vi "Main.vi"() -> ()   [LabVIEW 2023]
uses:
  3e66f978-0bac-48a9-bd70-621d12ad9d2c.vi
  <vilib>/JDP Science/JSONtext/JSON text to Variant.vi
  <vilib>/JDP Science/JSONtext/LVClass Serializer/JSONtext LVClass Serializer.lvclass
panel:
  out "error out":errorcluster
  in  "error in (no error)":errorcluster
  out "Find Json Files":path[](array[path])
  out "Array":T1(array[cluster])
  in  "取得するType名":string
  out "All Files in Dir":path[](array[path])
  in  "取得するフォルダのパス":path
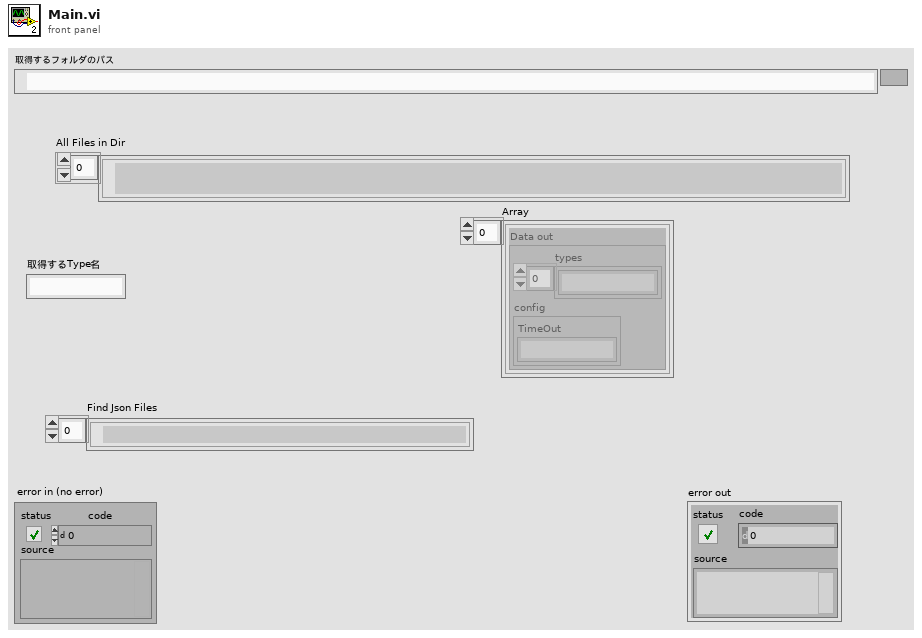
[diagram p1: front panel]
types:
  T1 = cluster{"Data out":cluster{"types":string[], "config":cluster{"TimeOut":string}}}[]
  T2 = cluster{"types":string[], "config":cluster{"TimeOut":string}}
  T3 = cluster{"Data out":cluster{"types":string[], "config":cluster{"TimeOut":string}}}
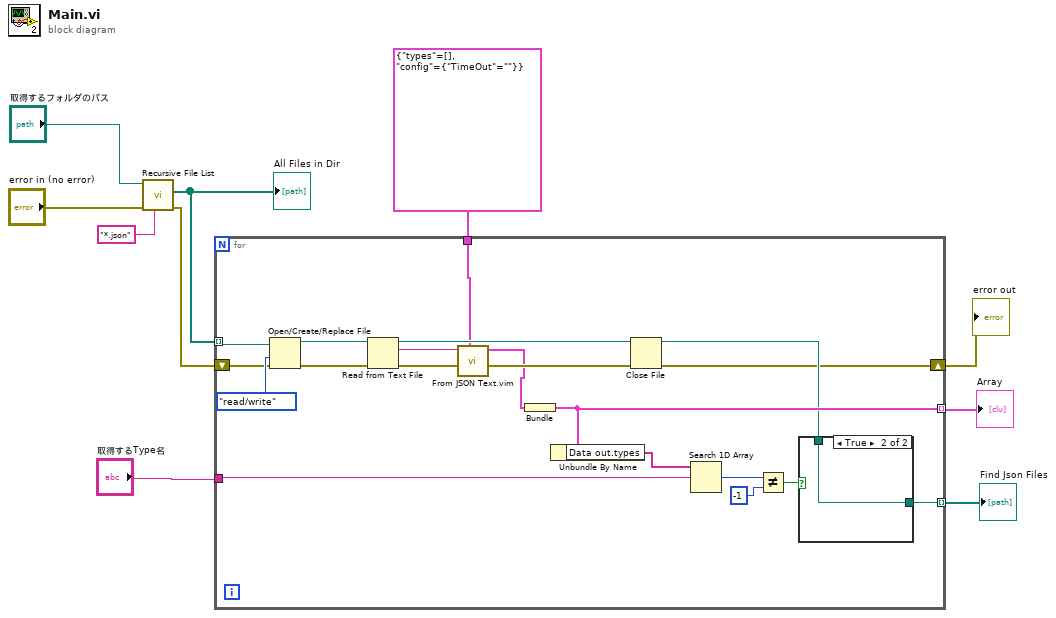
[diagram p0: block diagram]
diagram:
  n1 = call <vilib>:"Recursive File List.vi"("pattern"="*.json", "error in (no error)"="error in (no error)", "Folder Path"="取得するフォルダのパス") -> ("error out"=w7:errorcluster, "All Files in Dir"=w8:path[])  [unwired: 4 in, 3 out]
  "All Files in Dir" <- w8
  n2 = for {
    tunnel: w8 -> [w30] mode=indexing
    tunnel: T2 {"types"=[], "config"={"TimeOut"=""}} -> [w20]
    tunnel: [w19] -> w5 mode=indexing
    tunnel: "取得するType名" -> [w17]
    tunnel: [w13] -> w3 mode=indexing
    shift-right: [w11] -> w1
    shift-left: w7 -> [w26]
    n3 = Open/Create/Replace File(file path (use dialog)=w30, error in=w26, access (0:read/write)=enum16{"read/write", "read-only", "write-only"}."read/write") -> (refnum out=w28:refnum<file>, error out=w27:errorcluster)  [unwired: 3 in, 1 out]
    n4 = Read from Text File(file (use dialog)=w28, error in=w27) -> (refnum out=w22:refnum<file>, text=w25:string, error out=w24:errorcluster)  [unwired: 2 in, 1 out]
    n5 = call "From JSON Text.vim"("Data Type and Default Value"=w20, "error in (no error)"=w24, "JSON"=w25) -> ("error out"=w23:errorcluster, "Data out"=w21:T2)  [unwired: 7 in]
    n6 = Bundle("Data out"=w21) -> (w19:T3)  [unwired: 1 in]
    n7 = Unbundle By Name(w19) -> ("Data out.types"=w18:string[])
    n8 = Close File(refnum=w22, error in=w23) -> (path=w12:path, error out=w11:errorcluster)
    n9 = Search 1D Array(1D array=w18, element=w17) -> (index of element=w16:i32)  [unwired: 1 in]
    n10 = Not Equal?(x=w16, y=-1) -> (x != y?=w14:bool)
    n11 = case shown="True" w14 {
      tunnel: [_ w31] -> w13
      tunnel: w12 -> [_ w31]
      frame False {
      }
      frame True {
      }
    }
  }
  "Array" <- w5
  "Find Json Files" <- w3
  "error out" <- w1
